vi "ORS-ColorTable2ColorMapDataString.vi"(8 "reverse colormap?":bool, 9 "file path (dialog if empty)":path, 10 "Colormap (0 for file/array)":i32, 11 "colors (greymap if empty)":u32[](array[numeric])) -> (2 "colors output":u32[](array[numeric])=[0, 15728640, 64512, 15728640, 64512, 15728640, 63492, 15729664, 63492, 15729664, 62472, 15730688, 62472, 15730688, 61452, 15731712, 61452, 15731712, 60432, 15732736, 60432, 15732736, 59412, 15733760, 59412, 15733760, 58392, 15734784, 58392, 15734784, 57372, 15735808, 57372, 15735808, 56352, 15736832, 56352, 15736832, 55332, 15737856, 55332, 15737856, 54312, 15738880, 54312, 15738880, 53292, 15739904, 53292, 15739904, 52272, 15740928, 52272, 15740928, 51252, 15741952, 51252, 15741952, 50232, 15742976, 50232, 15742976, 49212, 15744000, 49212, 15744000, 48192, 15745024, 48192, 15745024, 47172, 15746048, 47172, 15746048, 46152, 15747072, 46152, 15747072, 45132, 15748096, 45132, 15748096, 44112, 15749120, 44112, 15749120, 43092, 16012288, 43092, 16012288, 42072, 16013312, 42072, 16013312, 41052, 16014336, 41052, 16014336, 40032, 16015360, 40032, 16015360, 39012, 16016384, 39012, 16016384, 37992, 16017408, 37992, 16017408, 36972, 16018432, 36972, 16018432, 35952, 16019456, 35952, 16019456, 34932, 16020480, 34932, 16020480, 33912, 16021504, 33912, 16021504, 32892, 16022528, 32892, 16022528, 31872, 16023552, 31872, 16023552, 30852, 16024576, 30852, 16024576, 29832, 16025600, 29832, 16025600, 28812, 16026624, 28812, 16026624, 27792, 16027648, 27792, 16027648, 26772, 16028672, 26772, 16028672, 25752, 16029696, 25752, 16029696, 24732, 16030720, 24732, 16030720, 23712, 16031744, 23712, 16031744, 22692, 16032768, 22692, 16032768, 21672, 16295936, 21672, 16295936, 20652, 16296960, 20652, 16296960, 19632, 16297984, 19632, 16297984, 18612, 16299008, 18612, 16299008, 17592, 16300032, 17592, 16300032, 16572, 16301056, 16572, 16301056, 15552, 16302080, 15552, 16302080, 14532, 16303104, 14532, 16303104, 13512, 16304128, 13512, 16304128, 12492, 16305152, 12492, 16305152, 11472, 16306176, 11472, 16306176, 10452, 16307200, 10452, 16307200, 9432, 16308224, 9432, 16308224, 8412, 16309248, 8412, 16309248, 7392, 16310272, 7392, 16310272, 6372, 16311296, 6372, 16311296, 5352, 16312320, 5352, 16312320, 4332, 16313344, 4332, 16313344, 3312, 16314368, 3312, 16314368, 2292, 16315392, 2292, 16315392, 1272, 16316416, 1272, 16579584, 16547840, 32896], 3 "colormap data string":string)   [LabVIEW 2021]
panel:
  out "color #":i32
  out "text":string="  0 128 128"
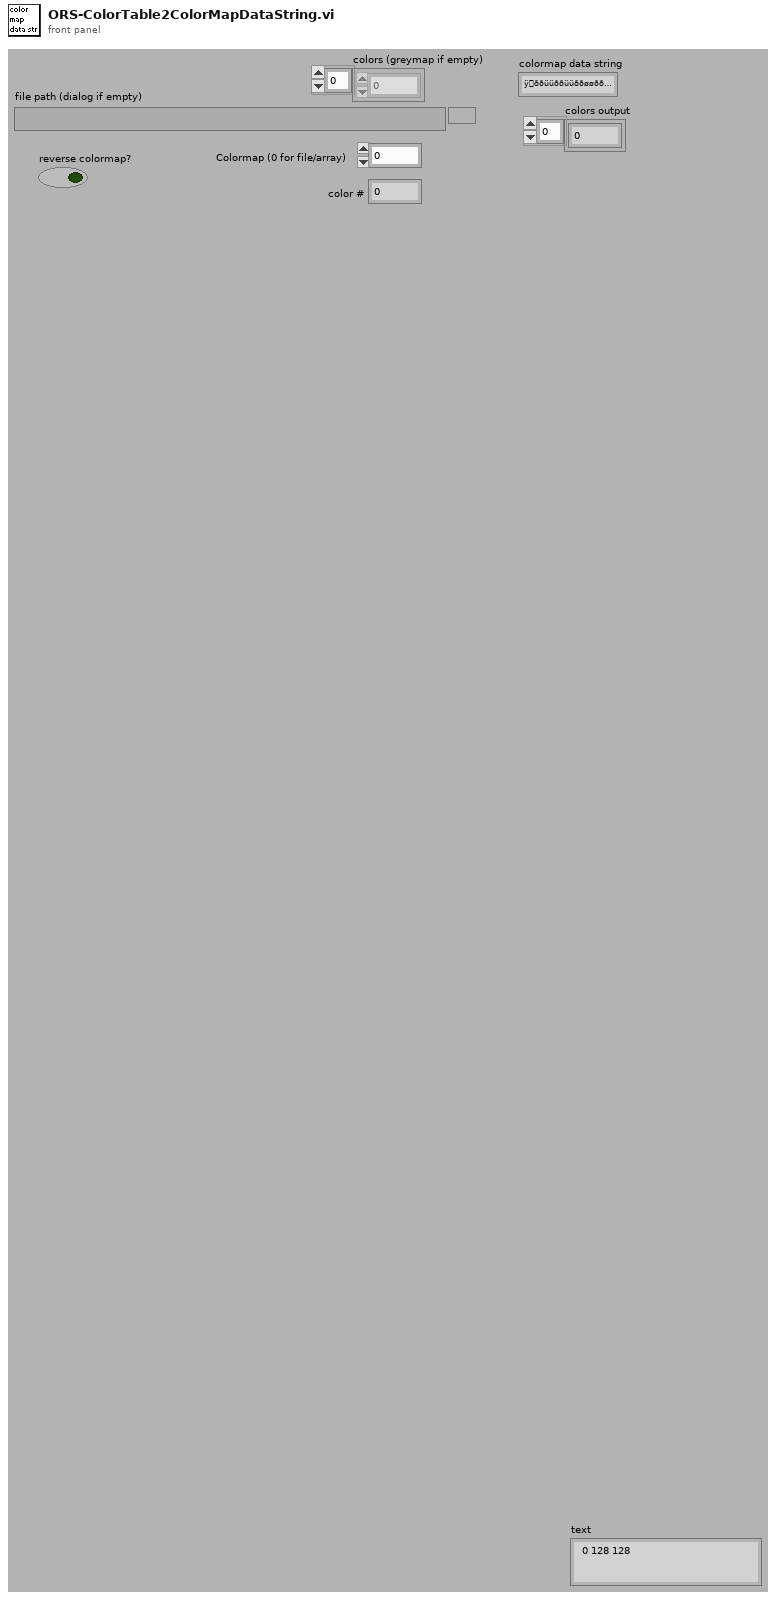
[diagram p1: front panel]
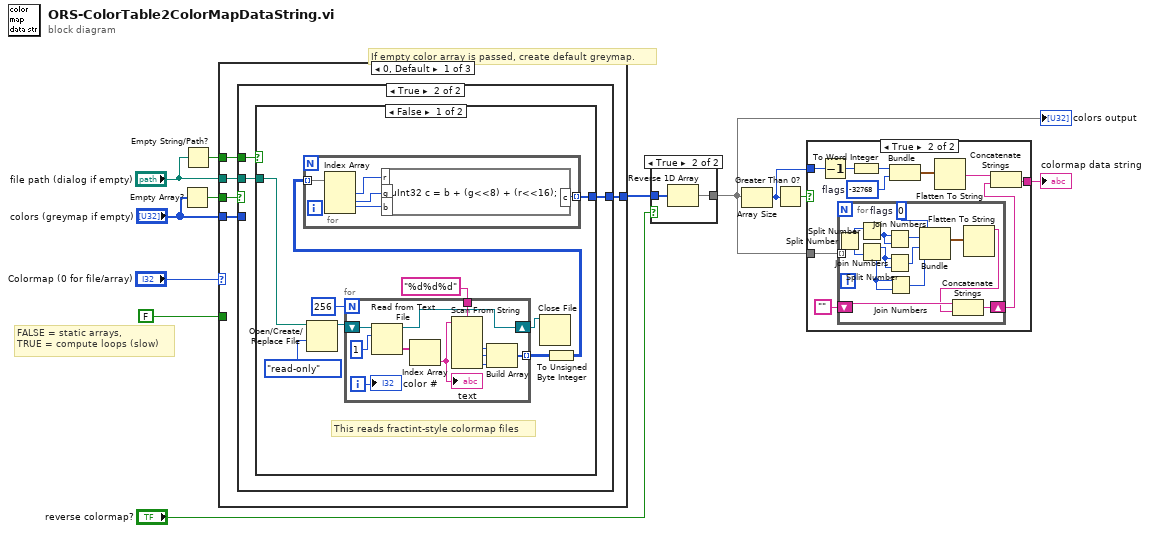
[diagram p0: block diagram]
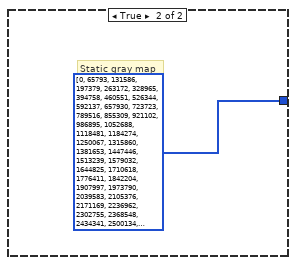
[diagram p4: hidden frame]
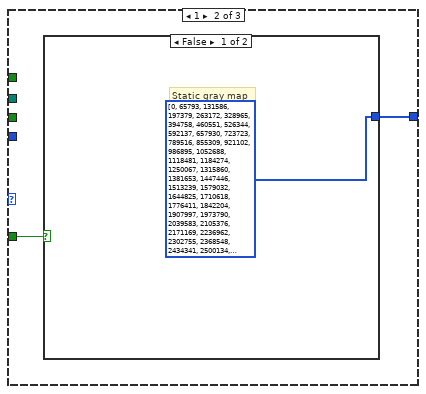
[diagram p5: hidden frame]
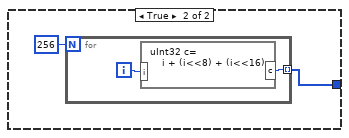
[diagram p6: hidden frame]
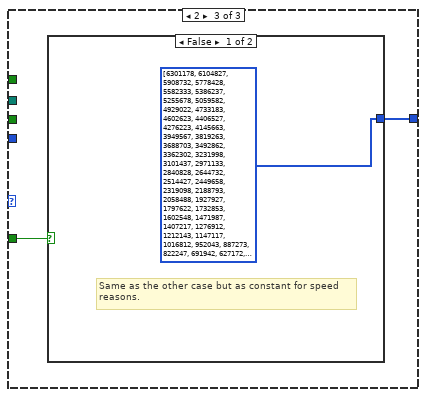
[diagram p7: hidden frame]
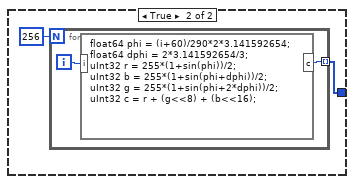
[diagram p8: hidden frame]
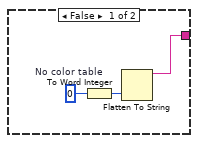
[diagram p9: hidden frame]
diagram:
  # "FALSE = static arrays,\nTRUE = compute loops (slow)"
  # "If empty color array is passed, create default greymap."
  n1 = Empty Array?(array="colors (greymap if empty)") -> (empty?=w8:bool)
  n2 = Empty String/Path?(string/path="file path (dialog if empty)") -> (empty?=w6:bool)
  n3 = case shown="0, Default" "Colormap (0 for file/array)" {
    tunnel: w8 -> [w17 _ _]
    tunnel: [w16 w48 w55] -> w3
    tunnel: "colors (greymap if empty)" -> [w15 _ _]
    tunnel: w6 -> [w14 _ _]
    tunnel: "file path (dialog if empty)" -> [w13 _ _]
    tunnel: FALSE -> [_ w49 w56]
    frame 0, Default {
      n4 = case shown="True" w17 {
        tunnel: [w18 w21] -> w16
        tunnel: w15 -> [w18 _]
        tunnel: w14 -> [_ w20]
        tunnel: w13 -> [_ w19]
        frame False {
        }
        frame True {
          n5 = case shown="False" w20 {
            tunnel: [w23 u32[] [0, 65793, 131586, 197379, 263172, 328965, 394758, 460551, 526344, 592137, 657930, 723723, 789516, 855309, 921102, 986895, 1052688, 1118481, 1184274, 1250067, 1315860, 1381653, 1447446, 1513239, 1579032, 1644825, 1710618, 1776411, 1842204, 1907997, 1973790, 2039583, 2105376, 2171169, 2236962, 2302755, 2368548, 2434341, 2500134, 2565927, 2631720, 2697513, 2763306, 2829099, 2894892, 2960685, 3026478, 3092271, 3158064, 3223857, 3289650, 3355443, 3421236, 3487029, 3552822, 3618615, 3684408, 3750201, 3815994, 3881787, 3947580, 4013373, 4079166, 4144959, 4210752, 4276545, 4342338, 4408131, 4473924, 4539717, 4605510, 4671303, 4737096, 4802889, 4868682, 4934475, 5000268, 5066061, 5131854, 5197647, 5263440, 5329233, 5395026, 5460819, 5526612, 5592405, 5658198, 5723991, 5789784, 5855577, 5921370, 5987163, 6052956, 6118749, 6184542, 6250335, 6316128, 6381921, 6447714, 6513507, 6579300, 6645093, 6710886, 6776679, 6842472, 6908265, 6974058, 7039851, 7105644, 7171437, 7237230, 7303023, 7368816, 7434609, 7500402, 7566195, 7631988, 7697781, 7763574, 7829367, 7895160, 7960953, 8026746, 8092539, 8158332, 8224125, 8289918, 8355711, 8421504, 8487297, 8553090, 8618883, 8684676, 8750469, 8816262, 8882055, 8947848, 9013641, 9079434, 9145227, 9211020, 9276813, 9342606, 9408399, 9474192, 9539985, 9605778, 9671571, 9737364, 9803157, 9868950, 9934743, 10000536, 10066329, 10132122, 10197915, 10263708, 10329501, 10395294, 10461087, 10526880, 10592673, 10658466, 10724259, 10790052, 10855845, 10921638, 10987431, 11053224, 11119017, 11184810, 11250603, 11316396, 11382189, 11447982, 11513775, 11579568, 11645361, 11711154, 11776947, 11842740, 11908533, 11974326, 12040119, 12105912, 12171705, 12237498, 12303291, 12369084, 12434877, 12500670, 12566463, 12632256, 12698049, 12763842, 12829635, 12895428, 12961221, 13027014, 13092807, 13158600, 13224393, 13290186, 13355979, 13421772, 13487565, 13553358, 13619151, 13684944, 13750737, 13816530, 13882323, 13948116, 14013909, 14079702, 14145495, 14211288, 14277081, 14342874, 14408667, 14474460, 14540253, 14606046, 14671839, 14737632, 14803425, 14869218, 14935011, 15000804, 15066597, 15132390, 15198183, 15263976, 15329769, 15395562, 15461355, 15527148, 15592941, 15658734, 15724527, 15790320, 15856113, 15921906, 15987699, 16053492, 16119285, 16185078, 16250871, 16316664, 16382457, 16448250, 16514043, 16579836, 16645629, 16711422, 16777215] ("Array")] -> w21
            tunnel: w19 -> [w24 _]
            frame False {
              # "This reads fractint-style colormap files"
              n6 = Open/Create/Replace File(file path (use dialog)=w24, access (0:read/write)=enum16{"read/write", "read-only", "write-only"}."read-only") -> (refnum out=w26:refnum<file>)  [unwired: 4 in, 2 out]
              n7 = for {
                N: 256 -> [_]
                shift-right: [w38] -> w28
                shift-left: w26 -> [w39]
                tunnel: "%d%d%d" ("format (%d)") -> [w45]
                tunnel: [w46] -> w29 mode=indexing
                i -> [w41]
                n8 = Read from Text File(file (use dialog)=w39, count=1) -> (refnum out=w38:refnum<file>, text=w37:string[])  [unwired: 2 in, 2 out]
                n9 = Index Array(array=w37) -> (element=w36:string)  [unwired: 1 in]
                "text" <- w36
                n10 = Scan From String(format string=w45, input string=w36) -> (output 1=w44:i32, output 2=w43:i32, output 3=w42:i32)  [unwired: 5 in, 3 out]
                n11 = Build Array(w44, w43, w42) -> (w46:i32[])
                "color #" <- w41
              }
              n12 = Close File(refnum=w28) -> ()  [unwired: 1 in, 2 out]
              n13 = To Unsigned Byte Integer(number=w29) -> (unsigned 8bit integer=w22:u8[][])
              n14 = for {
                tunnel: w22 -> [w35] mode=indexing
                tunnel: [w34] -> w23 mode=indexing
                n15 = Index Array(array=w35) -> (element #1=w33:u8, element #2=w32:u8, element #3=w31:u8)  [unwired: 3 in]
                n16 = formula code="uInt32 c = b + (g<<8) + (r<<16);"("r"=w33, "g"=w32, "b"=w31) -> ("c"=w34:u32)
              }
            }
            frame True {
              # "Static gray map"
            }
          }
        }
      }
    }
    frame 1 {
      n17 = case shown="False" w49 {
        tunnel: [u32[] [0, 65793, 131586, 197379, 263172, 328965, 394758, 460551, 526344, 592137, 657930, 723723, 789516, 855309, 921102, 986895, 1052688, 1118481, 1184274, 1250067, 1315860, 1381653, 1447446, 1513239, 1579032, 1644825, 1710618, 1776411, 1842204, 1907997, 1973790, 2039583, 2105376, 2171169, 2236962, 2302755, 2368548, 2434341, 2500134, 2565927, 2631720, 2697513, 2763306, 2829099, 2894892, 2960685, 3026478, 3092271, 3158064, 3223857, 3289650, 3355443, 3421236, 3487029, 3552822, 3618615, 3684408, 3750201, 3815994, 3881787, 3947580, 4013373, 4079166, 4144959, 4210752, 4276545, 4342338, 4408131, 4473924, 4539717, 4605510, 4671303, 4737096, 4802889, 4868682, 4934475, 5000268, 5066061, 5131854, 5197647, 5263440, 5329233, 5395026, 5460819, 5526612, 5592405, 5658198, 5723991, 5789784, 5855577, 5921370, 5987163, 6052956, 6118749, 6184542, 6250335, 6316128, 6381921, 6447714, 6513507, 6579300, 6645093, 6710886, 6776679, 6842472, 6908265, 6974058, 7039851, 7105644, 7171437, 7237230, 7303023, 7368816, 7434609, 7500402, 7566195, 7631988, 7697781, 7763574, 7829367, 7895160, 7960953, 8026746, 8092539, 8158332, 8224125, 8289918, 8355711, 8421504, 8487297, 8553090, 8618883, 8684676, 8750469, 8816262, 8882055, 8947848, 9013641, 9079434, 9145227, 9211020, 9276813, 9342606, 9408399, 9474192, 9539985, 9605778, 9671571, 9737364, 9803157, 9868950, 9934743, 10000536, 10066329, 10132122, 10197915, 10263708, 10329501, 10395294, 10461087, 10526880, 10592673, 10658466, 10724259, 10790052, 10855845, 10921638, 10987431, 11053224, 11119017, 11184810, 11250603, 11316396, 11382189, 11447982, 11513775, 11579568, 11645361, 11711154, 11776947, 11842740, 11908533, 11974326, 12040119, 12105912, 12171705, 12237498, 12303291, 12369084, 12434877, 12500670, 12566463, 12632256, 12698049, 12763842, 12829635, 12895428, 12961221, 13027014, 13092807, 13158600, 13224393, 13290186, 13355979, 13421772, 13487565, 13553358, 13619151, 13684944, 13750737, 13816530, 13882323, 13948116, 14013909, 14079702, 14145495, 14211288, 14277081, 14342874, 14408667, 14474460, 14540253, 14606046, 14671839, 14737632, 14803425, 14869218, 14935011, 15000804, 15066597, 15132390, 15198183, 15263976, 15329769, 15395562, 15461355, 15527148, 15592941, 15658734, 15724527, 15790320, 15856113, 15921906, 15987699, 16053492, 16119285, 16185078, 16250871, 16316664, 16382457, 16448250, 16514043, 16579836, 16645629, 16711422, 16777215] ("Array") w51] -> w48
        frame False {
          # "Static gray map"
        }
        frame True {
          n18 = for {
            N: 256 -> [_]
            tunnel: [w53] -> w51 mode=indexing
            i -> [w54]
            n19 = formula code="uInt32 c=\n    i + (i<<8) + (i<<16);"("i"=w54) -> ("c"=w53:u32)
          }
        }
      }
    }
    frame 2 {
      n20 = case shown="False" w56 {
        tunnel: [u32[] [6301178, 6104827, 5908732, 5778428, 5582333, 5386237, 5255678, 5059582, 4929022, 4733183, 4602623, 4406527, 4276223, 4145663, 3949567, 3819263, 3688703, 3492862, 3362302, 3231998, 3101437, 2971133, 2840828, 2644732, 2514427, 2449658, 2319098, 2188793, 2058488, 1927927, 1797622, 1732853, 1602548, 1471987, 1407217, 1276912, 1212143, 1147117, 1016812, 952043, 887273, 822247, 691942, 627172, 562402, 497377, 498143, 433373, 368347, 303577, 238807, 239317, 174547, 175313, 110287, 111053, 111562, 46792, 47302, 48068, 48577, 49343, 49852, 50362, 51128, 117173, 117683, 118192, 184493, 185003, 251048, 251558, 317603, 318112, 384158, 450203, 515992, 582037, 648083, 714128, 779917, 845963, 912008, 977797, 1109378, 1175167, 1240957, 1372538, 1438327, 1569652, 1700978, 1766767, 1898092, 2029418, 2160743, 2226532, 2357857, 2489183, 2620252, 2751577, 2882647, 3013972, 3145042, 3341903, 3472972, 3604042, 3735367, 3931973, 4063043, 4194112, 4390718, 4521787, 4718393, 4849463, 5045813, 5176882, 5373488, 5504302, 5700908, 5897258, 6028328, 6224678, 6421028, 6551842, 6748192, 6944798, 7075613, 7271963, 7468313, 7664408, 7795222, 7991572, 8187923, 8384018, 8514832, 8711183, 8907278, 9103628, 9234187, 9430282, 9626633, 9822728, 9953287, 10149382, 10345477, 10476037, 10672388, 10868483, 10998787, 11194882, 11390978, 11521537, 11717633, 11848193, 12044032, 12174592, 12370688, 12500992, 12631552, 12827648, 12957952, 13088512, 13284353, 13414913, 13545217, 13675778, 13806082, 13936387, 14132483, 14262788, 14327557, 14458117, 14588422, 14718727, 14849288, 14979593, 15044362, 15174667, 15305228, 15369998, 15500303, 15565072, 15630098, 15760403, 15825172, 15889942, 15954968, 16085273, 16150043, 16214813, 16279838, 16279072, 16343842, 16408868, 16473638, 16538408, 16537898, 16602668, 16601902, 16666928, 16666162, 16665653, 16730423, 16729913, 16729147, 16728638, 16727872, 16727363, 16726853, 16726087, 16660042, 16659532, 16659023, 16592722, 16592212, 16526167, 16525657, 16459612, 16459103, 16393057, 16327012, 16261223, 16195178, 16129132, 16063087, 15997298, 15931252, 15865207, 15799418, 15667837, 15602048, 15536258, 15404677, 15338888, 15207563, 15076237, 15010448, 14879123, 14747797, 14616472, 14550683, 14419358, 14288032, 14156963, 14025638, 13894568, 13763243, 13632173, 13435312, 13304243, 13173173, 13041848, 12845242, 12714172, 12583103, 12386497] ("Array") w58] -> w55
        frame False {
          # "Same as the other case but as constant for speed\nreasons."
        }
        frame True {
          n21 = for {
            N: 256 -> [_]
            tunnel: [w60] -> w58 mode=indexing
            i -> [w61]
            n22 = formula code="float64 phi = (i+60)/290*2*3.141592654;\nfloat64 dphi = 2*3.141592654/3;\nuInt32 r = 255*(1+sin(phi))/2;\nuInt32 b = 255*(1+sin(phi+dphi))/2;\nuInt32 g = 255*(1+sin(phi+2*dphi))/2;\nuInt32 c = r + (g<<8) + (b<<16);"("i"=w61) -> ("c"=w60:u32)
          }
        }
      }
    }
  }
  n23 = case shown="True" "reverse colormap?" {
    tunnel: w3 -> [w62 w64]
    tunnel: [w62 w63] -> w2
    frame False {
    }
    frame True {
      n24 = Reverse 1D Array(array=w64) -> (reversed array=w63:u32[])
    }
  }
  "colors output" <- w2
  n25 = Array Size(array=w2) -> (size(s)=w12:i32)
  n26 = Greater Than 0?(x=w12) -> (x > 0?=w11:bool)
  n27 = case shown="True" w11 {
    tunnel: w2 -> [_ w68]
    tunnel: w12 -> [_ w77]
    tunnel: [w65 w72] -> w10
    frame False {
      w67 = 0  # No color table
      n28 = To Word Integer(number=w67) -> (16bit integer=w66:i16)
      n29 = Flatten To String(anything=w66) -> (data string=w65:string)  [unwired: 3 in, 2 out]
    }
    frame True {
      w75 = i16 -32768  # flags
      n30 = Decrement(x=w77) -> (x-1=w69:i32)
      n31 = for {
        tunnel: w68 -> [w89] mode=indexing
        shift-right: [w86] -> w70
        shift-left: "" -> [w87]
        w88 = i16 0  # flags
        n32 = Split Number(x=w89) -> (hi(x)=w91:u16, lo(x)=w90:u16)
        n33 = Split Number(x=w91) -> (lo(x)=w78:u8)  [unwired: 1 out]
        n34 = Split Number(x=w90) -> (hi(x)=w84:u8, lo(x)=w83:u8)
        n35 = Join Numbers(hi=w78, lo=w78) -> ((hi.lo)=w85:u16)
        n36 = Join Numbers(hi=w84, lo=w84) -> ((hi.lo)=w82:u16)
        n37 = Join Numbers(hi=w83, lo=w83) -> ((hi.lo)=w81:u16)
        n38 = Bundle("flags"=w88, w85, w82, w81) -> (w80:cluster{"flags":i16, u16, u16, u16})  [unwired: 1 in]
        n39 = Flatten To String(anything=w80) -> (data string=w79:string)  [unwired: 3 in, 2 out]
        n40 = Concatenate Strings(w87, w79) -> (w86:string)
      }
      n41 = To Word Integer(number=w69) -> (16bit integer=w76:i16)
      n42 = Bundle(w76, "flags"=w75) -> (w74:cluster{i16, "flags":i16})  [unwired: 1 in]
      n43 = Flatten To String(anything=w74) -> (data string=w73:string)  [unwired: 3 in, 2 out]
      n44 = Concatenate Strings(w73, w70) -> (w72:string)
    }
  }
  "colormap data string" <- w10
